vi "Accident Detector.vi"() -> ()   [LabVIEW 2020]
panel:
  out "Boolean":bool
  out "Z":dbl(graph)
  out "Y":dbl(graph)
  out "X":dbl(graph)
  in  "VISA resource name":refnum<visa-resource-name>
  in  "Table Control":string[][](table)
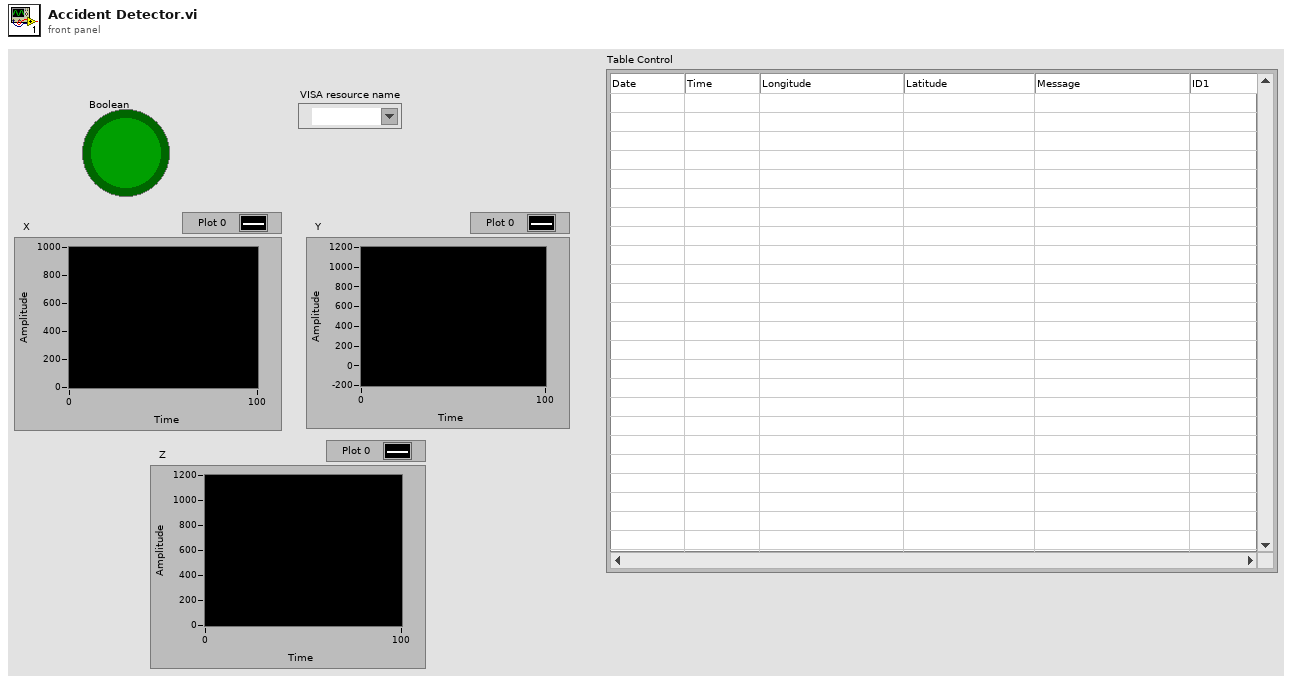
[diagram p1: front panel]
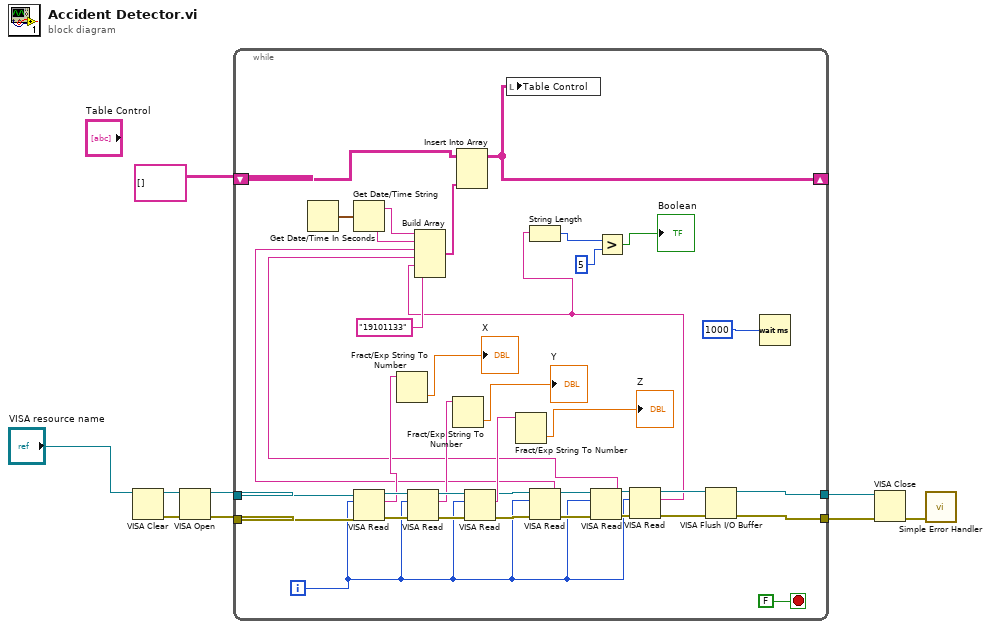
[diagram p0: block diagram]
diagram:
  n1 = VISA Clear(VISA resource name="VISA resource name") -> (VISA resource name out=w8:refnum<visa-resource-name>, error out=w9:errorcluster)  [unwired: 1 in]
  n2 = VISA Open(error in (no error)=w9, VISA resource name=w8) -> (VISA resource name=w7:refnum<visa-resource-name>, error out=w6:errorcluster)  [unwired: 3 in]
  n3 = while {
    tunnel: w7 -> [w32]
    tunnel: w6 -> [w31]
    shift-right: [w45] -> _
    shift-left: string[][] [] -> [w46]
    tunnel: [w39] -> w3
    tunnel: [w38] -> w1
    i -> [w15]
    stop <- FALSE stop-if-true
    n4 = Get Date/Time In Seconds() -> (seconds since 1Jan1904=w44:timestamp)
    n5 = Get Date/Time String(seconds (now)=w44) -> (date string=w43:string, time string=w42:string)  [unwired: 2 in]
    n6 = VISA Read(VISA resource name=w32, byte count=w15, error in (no error)=w31) -> (VISA resource name out=w36:refnum<visa-resource-name>, read buffer=w30:string, error out=w35:errorcluster)  [unwired: 1 out]
    n7 = Fract/Exp String To Number(string=w30) -> (number=→"X":dbl)  [unwired: 3 in, 1 out]
    n8 = VISA Read(VISA resource name=w36, byte count=w15, error in (no error)=w35) -> (VISA resource name out=w34:refnum<visa-resource-name>, read buffer=w29:string, error out=w33:errorcluster)  [unwired: 1 out]
    n9 = Fract/Exp String To Number(string=w29) -> (number=→"Y":dbl)  [unwired: 3 in, 1 out]
    n10 = VISA Read(VISA resource name=w34, byte count=w15, error in (no error)=w33) -> (VISA resource name out=w20:refnum<visa-resource-name>, read buffer=w25:string, error out=w19:errorcluster)  [unwired: 1 out]
    n11 = Fract/Exp String To Number(string=w25) -> (number=→"Z":dbl)  [unwired: 3 in, 1 out]
    n12 = VISA Read(VISA resource name=w20, byte count=w15, error in (no error)=w19) -> (VISA resource name out=w18:refnum<visa-resource-name>, read buffer=w16:string, error out=w17:errorcluster)  [unwired: 1 out]
    n13 = VISA Read(VISA resource name=w18, byte count=w15, error in (no error)=w17) -> (VISA resource name out=w24:refnum<visa-resource-name>, read buffer=w14:string, error out=w21:errorcluster)  [unwired: 1 out]
    n14 = VISA Read(VISA resource name=w24, byte count=w15, error in (no error)=w21) -> (VISA resource name out=w23:refnum<visa-resource-name>, read buffer=w13:string, error out=w22:errorcluster)  [unwired: 1 out]
    n15 = Build Array(w43, w42, w16, w14, w13, "19101133" ("element")) -> (w41:string[])
    n16 = Insert Into Array(array=w46, new element=w41) -> (w45:string[][])  [unwired: 2 in]
    n17 = local write "Table Control"(w45) -> ()
    n18 = String Length(string=w13) -> (length=w12:i32)
    n19 = Greater?(x=w12, y=5) -> (0:→"Boolean":bool)
    n20 = VISA Flush I/O Buffer(VISA resource name=w23, error in (no error)=w22) -> (VISA resource name out=w39:refnum<visa-resource-name>, error out=w38:errorcluster)  [unwired: 1 in]
    n21 = Wait (ms)(milliseconds to wait=u32 1000) -> ()  [unwired: 1 out]
  }
  n22 = VISA Close(VISA resource name=w3, error in (no error)=w1) -> (error out=w2:errorcluster)
  n23 = call <vilib>:"Simple Error Handler.vi"("error in (no error)"=w2) -> ()  [unwired: 4 in, 5 out]
